vi "Create ObjectBuffer.vi"(8 "error in":errorcluster, 10 "default":refnum<class>, 11 "bufSize":i32) -> (0 "error out":errorcluster, 3 "Buffer":refnum<data-value>)   [LabVIEW 2013, in "ObjectBuffer.lvclass"]
doc: "This VI creates a ring buffer of set size. This buffer is created in one place in the memory and is then accessed via pointer/reference.\n\nThe Data Type input is required because it defines the place in the memory to correct size thus removing the need for memory reallocation."
uses:
  ObjectBuffer.lvclass
  VariantBuffer/VariantBuffer.lvclass
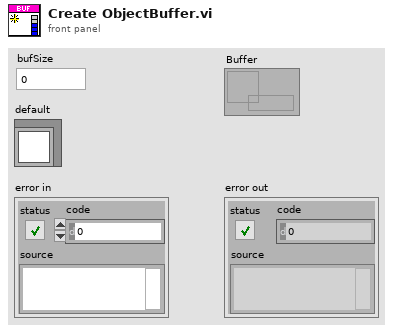
[diagram p1: front panel]
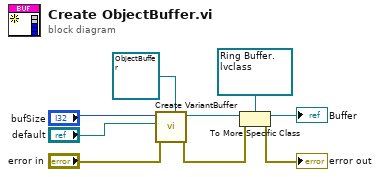
[diagram p0: block diagram]
diagram:
  n1 = call "Create VariantBuffer.vi"("Buffer"=refnum<class "ObjectBuffer.lvclass"> refnum ("Ring Buffer.lvclass"), "error in"="error in", "default"="default", "bufSize"="bufSize") -> ("error out"=w1:errorcluster, "Buffer"=w8:refnum<data-value>)  [unwired: 6 in]
  n2 = To More Specific Class(target class=refnum<data-value> refnum ("Buffer"), reference=w8, error in=w1) -> (specific class reference=→"Buffer":refnum<data-value>, error out=→"error out":errorcluster)
